vi "Get_Proj_Ref_Glob_From_File.vi"(2 "error in":errorcluster, 3 "Get default(?)":bool=TRUE, 4 "File Path":path=path "C:/Users/Marek/Desktop/LabView_Programs/QST_Proj/QST/Config_Files/project_reference_default.ini") -> (0 "error out":errorcluster, 1 "References":T1={"VI References"=[{"VI Name"="Channel_Map_Global", "String Path"="C:\\Users\\Daniel\\Desktop\\LabView\\QST\\Addons\\Arduino_Puls_Gen_Channel_Map\\Channel_Map_Global.vi"}, {"VI Name"="Set_Channel_Map", "String Path"="C:\\Users\\Daniel\\Desktop\\LabView\\QST\\Addons\\Arduino_Puls_Gen_Channel_Map\\Set_Channel_Map.vi"}, {"VI Name"="Sort_Channel_Map", "String Path"="C:\\Users\\Daniel\\Desktop\\LabView\\QST\\Addons\\Arduino_Puls_Gen_Channel_Map\\Sort_Channel_Map.vi"}, {"VI Name"="Prepare_Pulse_Seq", "String Path"="C:\\Users\\Daniel\\Desktop\\LabView\\QST\\Addons\\Prepare_Pulse_Sequence\\Prepare_Pulse_Seq.vi"}, {"VI Name"="Pulse_Sequence_Global", "String Path"="C:\\Users\\Daniel\\Desktop\\LabView\\QST\\Addons\\Prepare_Pulse_Sequence\\Pulse_Sequence_Global.vi"}, {"VI Name"="Set_Initial_Output_States", "String Path"="C:\\Users\\Daniel\\Desktop\\LabView\\QST\\Addons\\Prepare_Pulse_Sequence\\Set_Initial_Output_States.vi"}, {"VI Name"="Find_All_VIs", "String Path"="C:\\Users\\Daniel\\Desktop\\LabView\\QST\\Addons\\Project_Menager\\Find_All_VIs.vi"}, {"VI Name"="Open Project VI Reference 2012 NIVerified", "String Path"="C:\\Users\\Daniel\\Desktop\\LabView\\QST\\Addons\\Project_Menager\\Open Project VI Reference 2012 NIVerified.vi"}, {"VI Name"="Project_References_Global", "String Path"="C:\\Users\\Daniel\\Desktop\\LabView\\QST\\Addons\\Project_Menager\\Project_References_Global.vi"}, {"VI Name"="Tree", "String Path"="C:\\Users\\Daniel\\Desktop\\LabView\\QST\\Drivers\\Arduino_Pulse_Generator\\Tree.vi"}, {"VI Name"="Close", "String Path"="C:\\Users\\Daniel\\Desktop\\LabView\\QST\\Drivers\\Arduino_Pulse_Generator\\Close\\Close.vi"}, {"VI Name"="Pulse_Reset", "String Path"="C:\\Users\\Daniel\\Desktop\\LabView\\QST\\Drivers\\Arduino_Pulse_Generator\\Configurate\\Pulse_Reset.vi"}, {"VI Name"="Set_All_Outputs", "String Path"="C:\\Users\\Daniel\\Desktop\\LabView\\QST\\Drivers\\Arduino_Pulse_Generator\\Configurate\\Set_All_Outputs.vi"}, {"VI Name"="Set_Output_State", "String Path"="C:\\Users\\Daniel\\Desktop\\LabView\\QST\\Drivers\\Arduino_Pulse_Generator\\Configurate\\Set_Output_State.vi"}, {"VI Name"="Set_Pulse_Multiple_Channels", "String Path"="C:\\Users\\Daniel\\Desktop\\LabView\\QST\\Drivers\\Arduino_Pulse_Generator\\Configurate\\Set_Pulse_Multiple_Channels.vi"}, {"VI Name"="Set_Pulse_Single_Channel", "String Path"="C:\\Users\\Daniel\\Desktop\\LabView\\QST\\Drivers\\Arduino_Pulse_Generator\\Configurate\\Set_Pulse_Single_Channel.vi"}, {"VI Name"="Initialize", "String Path"="C:\\Users\\Daniel\\Desktop\\LabView\\QST\\Drivers\\Arduino_Pulse_Generator\\Initialize\\Initialize.vi"}, {"VI Name"="Run", "String Path"="C:\\Users\\Daniel\\Desktop\\LabView\\QST\\Drivers\\Arduino_Pulse_Generator\\Run\\Run.vi"}, {"VI Name"="Get_Unit", "String Path"="C:\\Users\\Daniel\\Desktop\\LabView\\QST\\Drivers\\Arduino_Pulse_Generator\\Utilize\\Get_Unit.vi"}, {"VI Name"="Identify", "String Path"="C:\\Users\\Daniel\\Desktop\\LabView\\QST\\Drivers\\Arduino_Pulse_Generator\\Utilize\\Identify.vi"}, {"VI Name"="Reset", "String Path"="C:\\Users\\Daniel\\Desktop\\LabView\\QST\\Drivers\\Arduino_Pulse_Generator\\Utilize\\Reset.vi"}, {"VI Name"="Set_Unit", "String Path"="C:\\Users\\Daniel\\Desktop\\LabView\\QST\\Drivers\\Arduino_Pulse_Generator\\Utilize\\Set_Unit.vi"}], "Global References"=[{"VI Name"="Channel_Map_Global", "String Path"="C:\\Users\\Daniel\\Desktop\\LabView\\QST\\Addons\\Arduino_Puls_Gen_Channel_Map\\Channel_Map_Global.vi"}, {"VI Name"="Pulse_Sequence_Global", "String Path"="C:\\Users\\Daniel\\Desktop\\LabView\\QST\\Addons\\Prepare_Pulse_Sequence\\Pulse_Sequence_Global.vi"}, {"VI Name"="Project_References_Global", "String Path"="C:\\Users\\Daniel\\Desktop\\LabView\\QST\\Addons\\Project_Menager\\Project_References_Global.vi"}], "INI References"=[{"VI Name"="Channel_Cluster", "String Path"="C:\\Users\\Daniel\\Desktop\\LabView\\QST\\Addons\\Arduino_Puls_Gen_Channel_Map\\Channel_Cluster.ctl"}, {"VI Name"="Channel_Pulse_Stream", "String Path"="C:\\Users\\Daniel\\Desktop\\LabView\\QST\\Drivers\\Arduino_Pulse_Generator\\Configurate\\Channel_Pulse_Stream.ctl"}], "CTL References"=[{"VI Name"="Channel_Cluster", "String Path"="C:\\Users\\Daniel\\Desktop\\LabView\\QST\\Addons\\Arduino_Puls_Gen_Channel_Map\\Channel_Cluster.ctl"}, {"VI Name"="Channel_Pulse_Stream", "String Path"="C:\\Users\\Daniel\\Desktop\\LabView\\QST\\Drivers\\Arduino_Pulse_Generator\\Configurate\\Channel_Pulse_Stream.ctl"}]})   [LabVIEW 2021]
uses:
  <vilib>/Utility/config.llb/Read Key (String).vi
  Project_References_Global.vi
  <vilib>/Utility/config.llb/NI_LVConfig.lvlib
panel:
  in  "Enum":T2(ring)=enum."VI Reference"
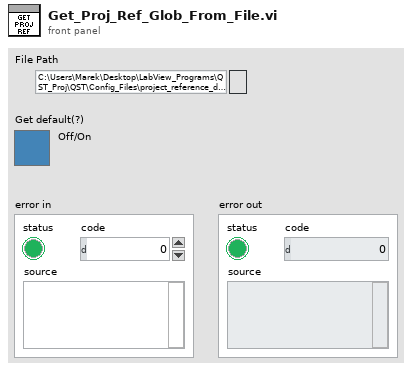
[diagram p1: front panel]
types:
  T1 = cluster{"VI References":cluster{"VI Name":string, "String Path":string}[], "Global References":cluster{"VI Name":string, "String Path":string}[], "INI References":cluster{"VI Name":string, "String Path":string}[], "CTL References":cluster{"VI Name":string, "String Path":string}[]}
  T2 = enum16{"Global Reference", "CLT Reference", "INI Reference", "VI Reference"}
  T3 = typedef "NI_LVConfig.lvlib/Config Data RefNum.ctl" = refnum<k1>
  T4 = cluster{"VI Name":string, "String Path":string}[]
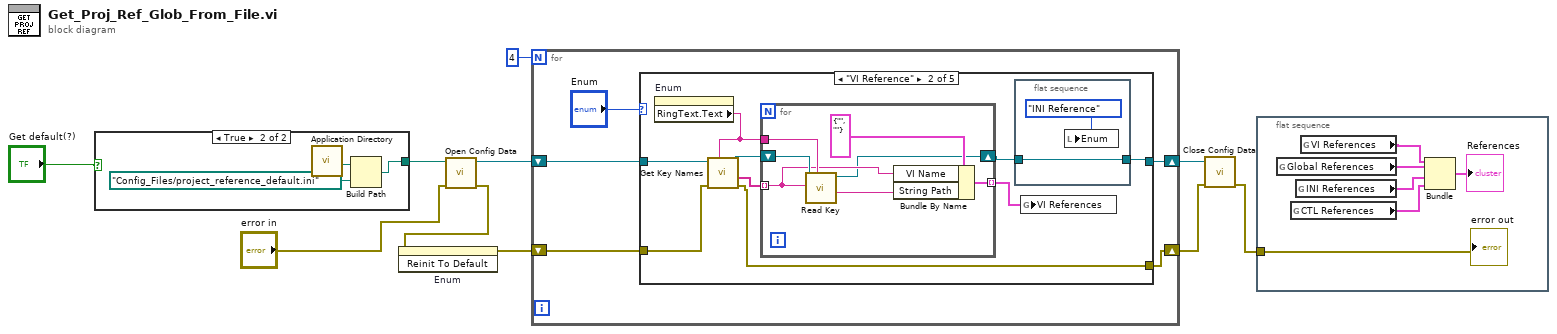
[diagram p0: block diagram]
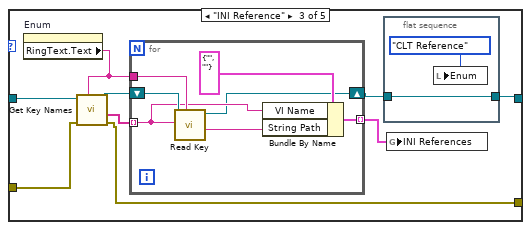
[diagram p3: hidden frame]
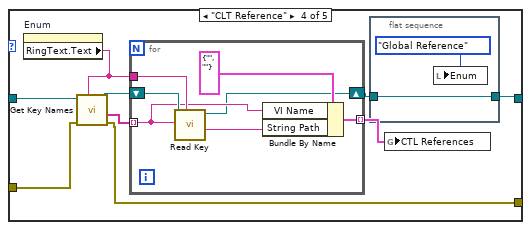
[diagram p4: hidden frame]
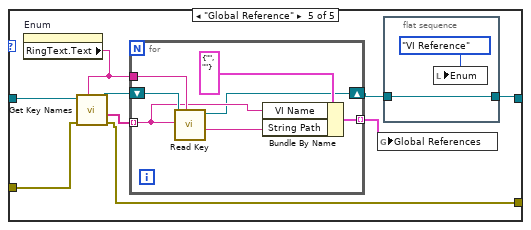
[diagram p5: hidden frame]
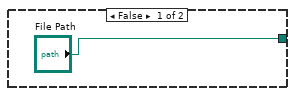
[diagram p6: hidden frame]
diagram:
  n1 = case shown="True" "Get default(?)" {
    tunnel: ["File Path" w12] -> w9
    frame False {
    }
    frame True {
      n2 = call <vilib>:"Application Directory.vi"() -> ("Application Directory"=w14:path)
      n3 = Build Path(base path=w14, name or relative path=path "Config_Files/project_reference_default.ini") -> (appended path=w12:path)
    }
  }
  n4 = call <vilib>:"Open Config Data.vi"("error in (no error)"="error in", "configuration file path"=w9) -> ("error out"=w3:errorcluster, "refnum"=w8:T3)  [unwired: 7 in, 1 out]
  n5 = invoke on="Enum" class="Enum (strict)" method="Reinit To Default"(error in=w3) -> (error out=w5:errorcluster)  [unwired: 2 in, 2 out]
  n6 = for {
    N: 4 -> [_]
    shift-right: [w18] -> w6
    shift-left: w8 -> [w19]
    shift-right: [w15] -> w2
    shift-left: w5 -> [w16]
    n7 = case shown="\"VI Reference\"" "Enum" {
      tunnel: w19 -> [w21 w30 w48 w66 w84]
      tunnel: [w21 w25 w43 w61 w79] -> w18
      tunnel: w16 -> [w20 w23 w41 w59 w77]
      tunnel: [w20 w22 w40 w58 w76] -> w15
      frame Default {
      }
      frame "VI Reference" {
        n8 = property on="Enum" class="Enum (strict)"() -> ("RingText.Text"=w26:string)  [unwired: 2 in, 2 out]
        n9 = call <vilib>:"Get Key Names.vi"("section"=w26, "error in (no error)"=w23, "refnum"=w30) -> ("error out"=w22:errorcluster, "key names"=w29:string[], "refnum out"=w28:T3)  [unwired: 5 in, 1 out]
        n10 = for {
          tunnel: w29 -> [w35] mode=indexing
          tunnel: w26 -> [w38]
          tunnel: [w34] -> w27 mode=indexing
          shift-right: [w33] -> w24
          shift-left: w28 -> [w39]
          n11 = call-poly <vilib>:"Read Key.vi"("section"=w38, "key"=w35, "refnum"=w39) -> ("value"=w36:string, "refnum out"=w33:T3)  [unwired: 5 in, 2 out]
          n12 = Bundle By Name(cluster=cluster{"VI Name":string, "String Path":string} {"VI Name"="", "String Path"=""} ("element"), "VI Name"=w35, "String Path"=w36) -> (w34:cluster{"VI Name":string, "String Path":string})
        }
        n13 = flat-sequence {
          tunnel: [w31] -> w25
          tunnel: w24 -> [w31]
          frame #0 {
            n14 = local write "Enum"(T2."INI Reference" ("Enum")) -> ()
          }
        }
        n15 = global write "Project_References_Global.vi" "VI References"(w27) -> ()
      }
      frame "INI Reference" {
        n16 = property on="Enum" class="Enum (strict)"() -> ("RingText.Text"=w44:string)  [unwired: 2 in, 2 out]
        n17 = call <vilib>:"Get Key Names.vi"("section"=w44, "error in (no error)"=w41, "refnum"=w48) -> ("error out"=w40:errorcluster, "key names"=w47:string[], "refnum out"=w46:T3)  [unwired: 5 in, 1 out]
        n18 = for {
          tunnel: w47 -> [w53] mode=indexing
          tunnel: w44 -> [w56]
          tunnel: [w52] -> w45 mode=indexing
          shift-right: [w51] -> w42
          shift-left: w46 -> [w57]
          n19 = call-poly <vilib>:"Read Key.vi"("section"=w56, "key"=w53, "refnum"=w57) -> ("value"=w54:string, "refnum out"=w51:T3)  [unwired: 5 in, 2 out]
          n20 = Bundle By Name(cluster=cluster{"VI Name":string, "String Path":string} {"VI Name"="", "String Path"=""} ("element"), "VI Name"=w53, "String Path"=w54) -> (w52:cluster{"VI Name":string, "String Path":string})
        }
        n21 = flat-sequence {
          tunnel: [w49] -> w43
          tunnel: w42 -> [w49]
          frame #0 {
            n22 = local write "Enum"(T2."CLT Reference" ("Enum")) -> ()
          }
        }
        n23 = global write "Project_References_Global.vi" "INI References"(w45) -> ()
      }
      frame "CLT Reference" {
        n24 = property on="Enum" class="Enum (strict)"() -> ("RingText.Text"=w62:string)  [unwired: 2 in, 2 out]
        n25 = call <vilib>:"Get Key Names.vi"("section"=w62, "error in (no error)"=w59, "refnum"=w66) -> ("error out"=w58:errorcluster, "key names"=w65:string[], "refnum out"=w64:T3)  [unwired: 5 in, 1 out]
        n26 = for {
          tunnel: w65 -> [w71] mode=indexing
          tunnel: w62 -> [w74]
          tunnel: [w70] -> w63 mode=indexing
          shift-right: [w69] -> w60
          shift-left: w64 -> [w75]
          n27 = call-poly <vilib>:"Read Key.vi"("section"=w74, "key"=w71, "refnum"=w75) -> ("value"=w72:string, "refnum out"=w69:T3)  [unwired: 5 in, 2 out]
          n28 = Bundle By Name(cluster=cluster{"VI Name":string, "String Path":string} {"VI Name"="", "String Path"=""} ("element"), "VI Name"=w71, "String Path"=w72) -> (w70:cluster{"VI Name":string, "String Path":string})
        }
        n29 = flat-sequence {
          tunnel: [w67] -> w61
          tunnel: w60 -> [w67]
          frame #0 {
            n30 = local write "Enum"(T2."Global Reference" ("Enum")) -> ()
          }
        }
        n31 = global write "Project_References_Global.vi" "CTL References"(w63) -> ()
      }
      frame "Global Reference" {
        n32 = property on="Enum" class="Enum (strict)"() -> ("RingText.Text"=w80:string)  [unwired: 2 in, 2 out]
        n33 = call <vilib>:"Get Key Names.vi"("section"=w80, "error in (no error)"=w77, "refnum"=w84) -> ("error out"=w76:errorcluster, "key names"=w83:string[], "refnum out"=w82:T3)  [unwired: 5 in, 1 out]
        n34 = for {
          tunnel: w83 -> [w89] mode=indexing
          tunnel: w80 -> [w92]
          tunnel: [w88] -> w81 mode=indexing
          shift-right: [w87] -> w78
          shift-left: w82 -> [w93]
          n35 = call-poly <vilib>:"Read Key.vi"("section"=w92, "key"=w89, "refnum"=w93) -> ("value"=w90:string, "refnum out"=w87:T3)  [unwired: 5 in, 2 out]
          n36 = Bundle By Name(cluster=cluster{"VI Name":string, "String Path":string} {"VI Name"="", "String Path"=""} ("element"), "VI Name"=w89, "String Path"=w90) -> (w88:cluster{"VI Name":string, "String Path":string})
        }
        n37 = global write "Project_References_Global.vi" "Global References"(w81) -> ()
        n38 = flat-sequence {
          tunnel: [w85] -> w79
          tunnel: w78 -> [w85]
          frame #0 {
            n39 = local write "Enum"(T2."VI Reference" ("Enum")) -> ()
          }
        }
      }
    }
  }
  n40 = call <vilib>:"Close Config Data.vi"("error in (no error)"=w2, "refnum"=w6) -> ("error out"=w1:errorcluster)  [unwired: 8 in, 1 out]
  n41 = flat-sequence {
    tunnel: w1 -> [w94]
    frame #0 {
      n42 = global read "Project_References_Global.vi" "Global References"() -> (w98:T4)
      n43 = global read "Project_References_Global.vi" "CTL References"() -> (w97:T4)
      n44 = global read "Project_References_Global.vi" "INI References"() -> (w95:T4)
      n45 = global read "Project_References_Global.vi" "VI References"() -> (w99:T4)
      n46 = Bundle("VI References"=w99, "Global References"=w98, "INI References"=w95, "CTL References"=w97) -> (→"References":T1)  [unwired: 1 in]
      "error out" <- w94
    }
  }
